vi "Z Aux Direct Move Circ Abs Sp.vi"(5 "idirection":i32, 6 "fcenter2":sgl, 7 "fcenter1":sgl, 8 "error in (no error)":errorcluster caption="错误输入（无错误）", 9 "fend2":sgl, 10 "fend1":sgl, 11 "handle":u32) -> (0 "error out":errorcluster caption="错误输出", 2 "function return":i32, 3 "handle out":u32)   [LabVIEW 2015, in "zauxdll.lvlib"]
doc: "int32 __stdcall ZAux_Direct_MoveCircAbsSp(ZMC_HANDLE handle, float fend1, float fend2, float fcenter1, float fcenter2, int idirection);"
uses:
  zauxdll.lvlib
  zauxdll.dll
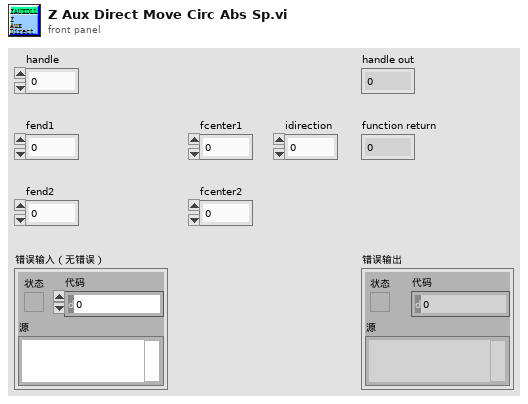
[diagram p1: front panel]
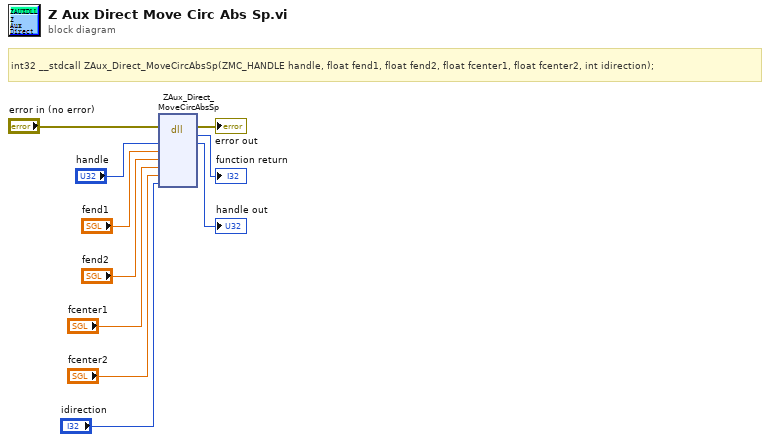
[diagram p0: block diagram]
diagram:
  # "int32 __stdcall ZAux_Direct_MoveCircAbsSp(ZMC_HANDLE handle, float fend1, float fend2, float fcenter1, float fcenter2, int idirection);"
  n1 = dll-call lib="C:/Users/VIC/Desktop/GOGORO_Oringnal - Panasonic/system/LLB/zmotion/zaux/zauxdll.*" fn="ZAux_Direct_MoveCircAbsSp"(error in="error in (no error)", "handle"="handle", "fend1"="fend1", "fend2"="fend2", "fcenter1"="fcenter1", "fcenter2"="fcenter2", "idirection"="idirection") -> (error out=→"error out":errorcluster, →"function return":i32, "handle"=→"handle out":u32)  [unwired: 7 in, 1 out]
